vi "Write Data File.vi"(8 "error in (no error)":errorcluster, 10 "Write Data File Arguments":T1, 11 "CSV Test Log in":refnum<class "CSV Test Log.lvclass">) -> (0 "error out":errorcluster, 2 "Relative Path":string, 3 "CSV Test Log out":refnum<class "CSV Test Log.lvclass">)   [LabVIEW 2015, in "CSV Test Log.lvclass"]
uses:
  CSV Test Log.lvclass
  Typedefs/Write Data File Arguments.ctl
  CSV Test Log.lvclass/CSV Test Log.ctl
  Typedefs/FAMT Typedefs.lvlib
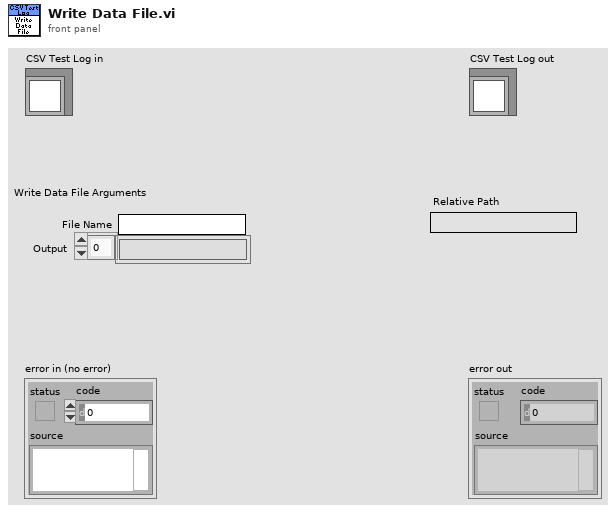
[diagram p1: front panel]
types:
  T1 = typedef "FAMT Typedefs.lvlib/Write Data File Arguments.ctl" = cluster{"File Name":string, "Output":string[]}
  T2 = enum16{"open", "replace", "create", "open or create", "replace or create", "replace or create with confirmation"}
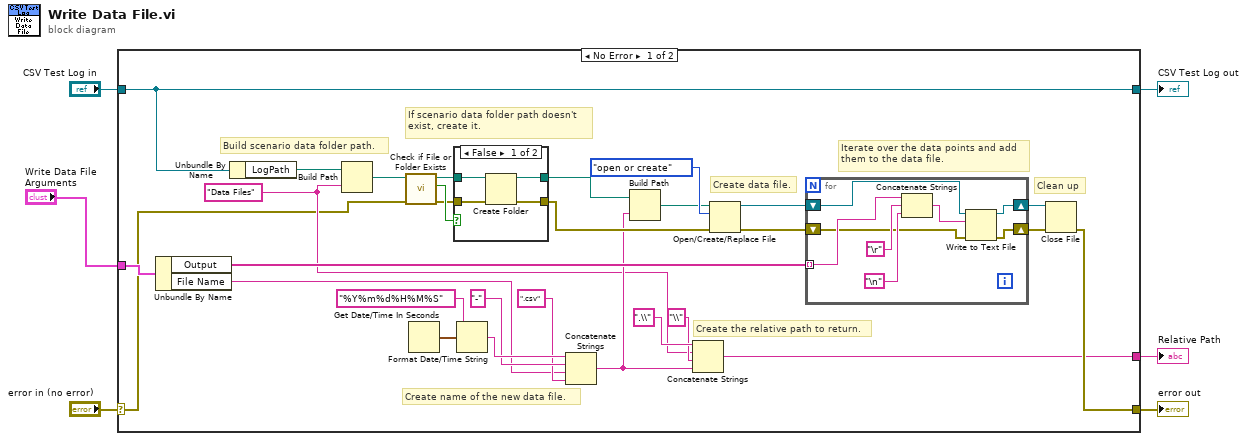
[diagram p0: block diagram]
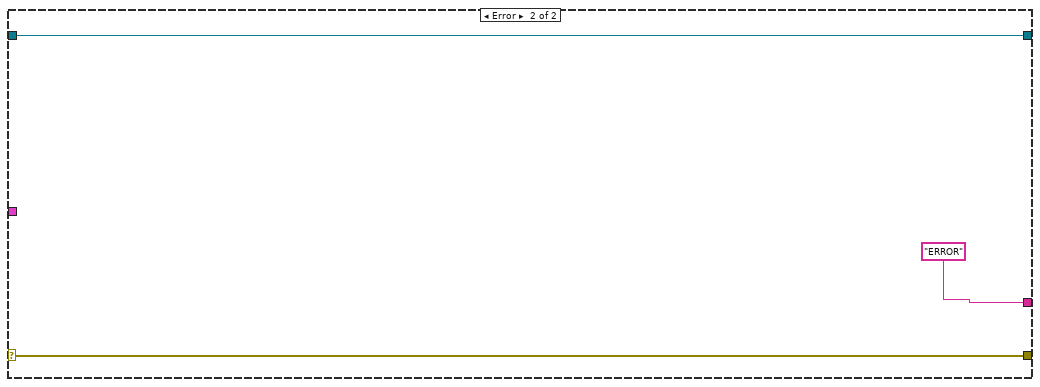
[diagram p3: hidden frame]
diagram:
  n1 = case shown="No Error" "error in (no error)" {
    selector: "error in (no error)" -> [w7 w52]
    tunnel: [w13 w52] -> w5
    tunnel: "CSV Test Log in" -> [w35 w51]
    tunnel: [w35 w51] -> w3
    tunnel: "Write Data File Arguments" -> [w29 _]
    tunnel: [w9 "ERROR"] -> w2
    frame No Error {
      w8 = "Data Files" ("format string")
      # "Clean up"
      # "Iterate over the data points and add\nthem to the data file."
      # "Create data file."
      # "Create the relative path to return."
      # "Create name of the new data file."
      # "If scenario data folder path doesn't\nexist, create it."
      # "Build scenario data folder path."
      n2 = Unbundle By Name(w29) -> ("Output"=w18:string[], "File Name"=w19:string)
      n3 = Unbundle By Name(w35) -> ("LogPath"=w31:path)
      n4 = Build Path(base path=w31, name or relative path=w8) -> (appended path=w30:path)
      n5 = call <vilib>:"Check if File or Folder Exists.vi"("error in (no error)"=w7, "path"=w30) -> ("error out"=w32:errorcluster, "file or folder exists?"=w34:bool, "dup path"=w33:path)  [unwired: 7 in]
      n6 = Get Date/Time In Seconds() -> (seconds since 1Jan1904=w25:timestamp)
      n7 = case shown="False" w34 {
        tunnel: w33 -> [w47 w49]
        tunnel: w32 -> [w46 w48]
        tunnel: [w45 w49] -> w28
        tunnel: [w44 w48] -> w21
        frame False {
          n8 = Create Folder(path (use dialog)=w47, error in=w46) -> (created path=w45:path, error out=w44:errorcluster)  [unwired: 1 in, 1 out]
        }
        frame True {
        }
      }
      n9 = Format Date/Time String(time format string (%c)="%Y%m%d%H%M%S", seconds (now)=w25) -> (date/time string=w27:string)  [unwired: 1 in]
      n10 = Concatenate Strings(w27, "-" ("string"), w19, ".csv" ("string")) -> (w10:string)
      n11 = Build Path(base path=w28, name or relative path=w10) -> (appended path=w20:path)
      n12 = Concatenate Strings(".\\" ("string"), w8, "\\" ("string"), w10) -> (w9:string)
      n13 = Open/Create/Replace File(file path (use dialog)=w20, error in=w21, operation (0:open)=T2."open or create") -> (refnum out=w17:refnum<file>, error out=w16:errorcluster)  [unwired: 3 in, 1 out]
      n14 = for {
        tunnel: w18 -> [w37] mode=indexing
        shift-right: [w39] -> w14
        shift-left: w16 -> [w36]
        shift-right: [w38] -> w15
        shift-left: w17 -> [w40]
        n15 = Concatenate Strings(w37, "\r", "\n") -> (w41:string)
        n16 = Write to Text File(file (use dialog)=w40, text=w41, error in=w36) -> (refnum out=w38:refnum<file>, error out=w39:errorcluster)  [unwired: 1 in, 1 out]
      }
      n17 = Close File(refnum=w15, error in=w14) -> (error out=w13:errorcluster)  [unwired: 1 out]
    }
    frame Error {
    }
  }
  "error out" <- w5
  "CSV Test Log out" <- w3
  "Relative Path" <- w2
